vi "Kinect Depth Controler.vi"() -> ()   [LabVIEW 2017]
uses:
  subVIs/Video Resolution Control.ctl
  subVIs/Video Format Control.ctl
  subVIs/Depth Format Control.ctl
  subVIs/Depth Resolution Control.ctl
  subVIs/Led Control.ctl
  subVIs/Log Level Control.ctl
panel:
  out "error out":errorcluster
  in  "Led Option":T1=enum."LED_RED"
  in  "Video & Depth Config":T6
  in  "Tilt degree":i32=5 min=-28 max=28
  in  "stop":bool
  out "Depth image":picture
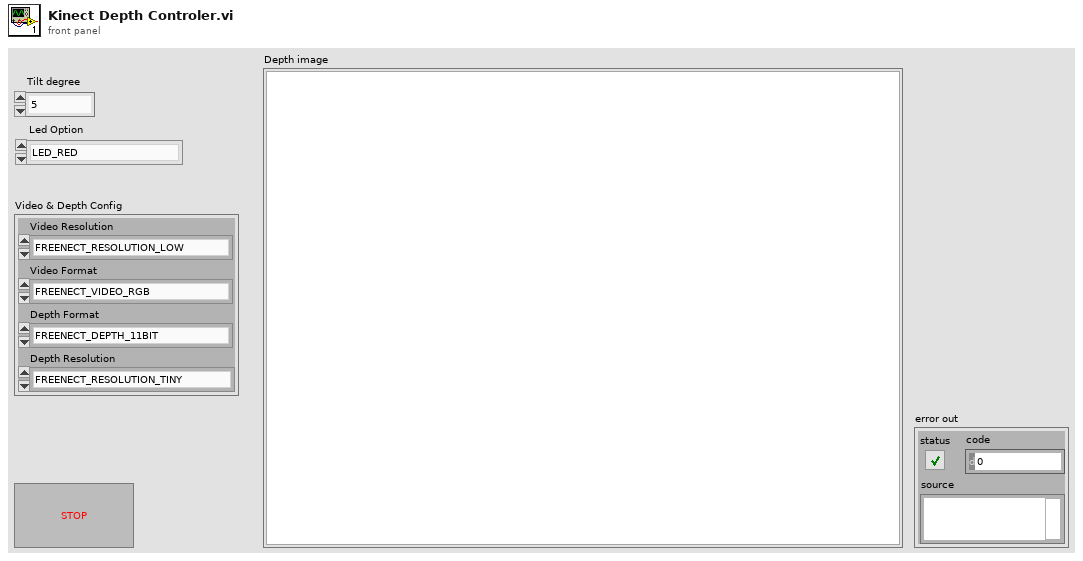
[diagram p1: front panel]
types:
  T1 = typedef "Led Control.ctl" = enum32{"LED_OFF", "LED_GREEN", "LED_RED", "LED_YELLOW", "LED_BLINK_GREEN", "LED_BLINK_GREEN2", "LED_BLINK_RED_YELLOW"}
  T2 = typedef "Video Resolution Control.ctl" = enum32{"FREENECT_RESOLUTION_LOW", "FREENECT_RESOLUTION_MEDIUM", "FREENECT_RESOLUTION_HIGH"}
  T3 = typedef "Video Format Control.ctl" = enum32{"FREENECT_VIDEO_RGB", "FREENECT_VIDEO_BAYER", "FREENECT_VIDEO_IR_8BIT", "FREENECT_VIDEO_IR_10BIT", "FREENECT_VIDEO_IR_10BIT_PACKED", "FREENECT_VIDEO_YUV_RGB", "FREENECT_VIDEO_YUV_RAW"}
  T4 = typedef "Depth Format Control.ctl" = enum32{"FREENECT_DEPTH_11BIT", "FREENECT_DEPTH_10BIT", "FREENECT_DEPTH_11BIT_PACKED", "FREENECT_DEPTH_10BIT_PACKED", "FREENECT_DEPTH_REGISTERED", "FREENECT_DEPTH_MM"}
  T5 = typedef "Depth Resolution Control.ctl" = enum16{"FREENECT_RESOLUTION_TINY", "FREENECT_RESOLUTION_LOW", "FREENECT_RESOLUTION_MEDIUM"}
  T6 = cluster{"Video Resolution":T2, "Video Format":T3, "Depth Format":T4, "Depth Resolution":T5}
  T7 = typedef "Log Level Control.ctl" = enum32{"FREENECT_LOG_FATAL", "FREENECT_LOG_ERROR", "FREENECT_LOG_WARNING", "FREENECT_LOG_NOTICE", "FREENECT_LOG_INFO", "FREENECT_LOG_DEBUG", "FREENECT_LOG_SPEW", "FREENECT_LOG_FLOOD"}
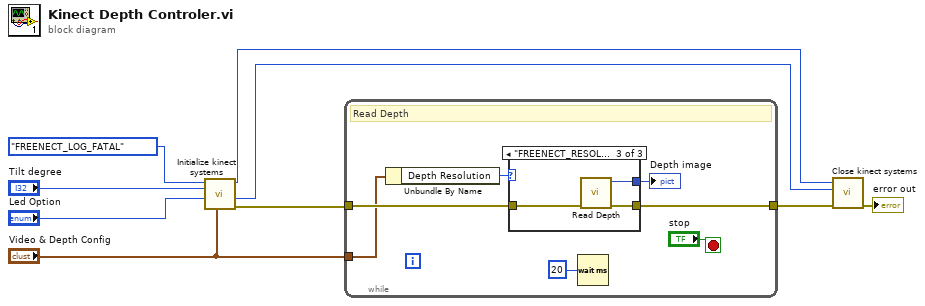
[diagram p0: block diagram]
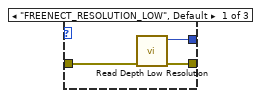
[diagram p2: hidden frame]
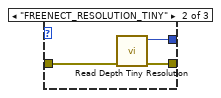
[diagram p3: hidden frame]
diagram:
  n1 = call "Initialize kinect systems.vi"("Video and Depth config"="Video & Depth Config", "Led Option"="Led Option", "tilt degree"="Tilt degree", "Log Level"=Log_Level_Control."FREENECT_LOG_FATAL") -> ("error out"=w8:errorcluster, "Kinect Handle"=w7:i64, "Video Handle out"=w1:i64)  [unwired: 4 in, 1 out]
  n2 = while {
    tunnel: w8 -> [w14]
    tunnel: [w13] -> w9
    tunnel: "Video & Depth Config" -> [w10]
    stop <- "stop" stop-if-true
    # "Read Depth"
    n3 = Unbundle By Name(w10) -> ("Depth Resolution"=w11:T5)
    n4 = case shown="\"FREENECT_RESOLUTION_MEDIUM\"" w11 {
      tunnel: w14 -> [w19 w20 w25]
      tunnel: [w18 w21 w24] -> w13
      tunnel: [w17 w22 w23] -> w12
      frame "FREENECT_RESOLUTION_LOW", Default {
        n5 = call "Read Depth Low Resolution.vi"("error in (no error)"=w19) -> ("error out"=w18:errorcluster, "Depth image"=w17:picture)  [unwired: 9 in]
      }
      frame "FREENECT_RESOLUTION_TINY" {
        n6 = call "Read Depth Tiny Resolution.vi"("error in (no error)"=w20) -> ("error out"=w21:errorcluster, "Depth image"=w22:picture)  [unwired: 9 in]
      }
      frame "FREENECT_RESOLUTION_MEDIUM" {
        n7 = call "Read Depth.vi"("error in (no error)"=w25) -> ("error out"=w24:errorcluster, "Depth image"=w23:picture)  [unwired: 9 in]
      }
    }
    "Depth image" <- w12
    n8 = Wait (ms)(milliseconds to wait=u32 20) -> ()  [unwired: 1 out]
  }
  n9 = call "Close kinect systems.vi"("error in (no error)"=w9, "Kinect Handle"=w7, "Video handle in"=w1) -> ("error out"=→"error out":errorcluster)  [unwired: 8 in]
